vi "Plugin.UDP.Set Connection IDs.vi"(10 "connection IDs":refnum<k16>[](array[refnum]), 11 "UDP Plugin in":refnum<class "UDP Plugin.lvclass">) -> (3 "UDP Plugin out":refnum<class "UDP Plugin.lvclass">)   [LabVIEW 2017, in "UDP Plugin.lvclass"]
uses:
  UDP Plugin.lvclass
  UDP Plugin.lvclass/UDP Plugin.ctl
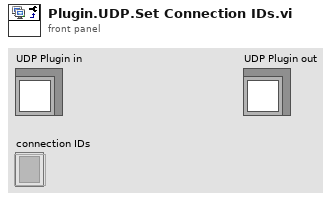
[diagram p1: front panel]
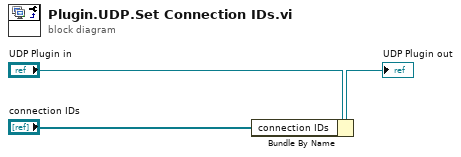
[diagram p0: block diagram]
diagram:
  n1 = Bundle By Name(cluster="UDP Plugin in", "connection IDs"="connection IDs") -> (→"UDP Plugin out":refnum<class "UDP Plugin.lvclass">)
